vi "Send Update Device Line Configuration.vi"(7 "Message Priority (Normal)":T3=enum."Normal", 8 "error in (no error)":errorcluster, 10 "Line Configuration":T1, 11 "Message Enqueuer":refnum<class "Message Enqueuer.lvclass">) -> (0 "error out":errorcluster, 3 "Message Enqueuer out":refnum<class "Message Enqueuer.lvclass">)   [LabVIEW 2016, in "Optimization Framework.lvlib" / "Update Device Line Configuration Msg.lvclass"]
doc: "This VI sends the message to an actor."
uses:
  Update Device Line Configuration Msg.lvclass
  <vilib>/ActorFramework/Message Enqueuer/Message Enqueuer.lvclass
  <vilib>/ActorFramework/Message Enqueuer/Message Priority.ctl
  Optimization/Controls/Optimization Parameters Line Configuration.ctl
  Optimization/Controls/Optimization Line Configuration Enum.ctl
  C:/Program Files (x86)/National Instruments/LabVIEW 2016/vi.lib/ActorFramework/Message/Message.lvclass
  Update Device Line Configuration Msg.lvclass/Update Device Line Configuration Msg.ctl
  <vilib>/ActorFramework/Message Enqueuer/Message Enqueuer.lvclass/Message Enqueuer.ctl
  <vilib>/ActorFramework/Message Priority Queue/Priority Enqueue.vi
  Optimization/Optimization.lvclass
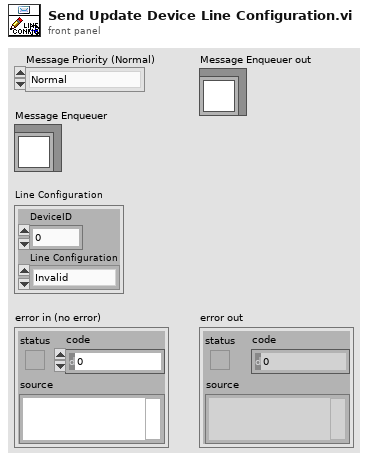
[diagram p1: front panel]
types:
  T1 = typedef "Optimization Framework.lvlib/Optimization.lvclass/Optimization Parameters Line Configuration.ctl" = cluster{"DeviceID":u64, "Line Configuration":T2}
  T2 = typedef "Optimization Framework.lvlib/Optimization.lvclass/Optimization Line Configuration Enum.ctl" = enum8{"Invalid", "L-L", "L-N", "L-G"}
  T3 = typedef "Actor Framework.lvlib/Message Enqueuer.lvclass/Message Priority.ctl" = enum16{"Low", "Normal", "High"}
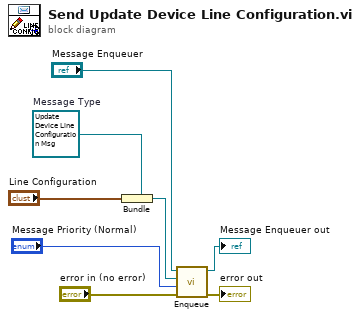
[diagram p0: block diagram]
diagram:
  w5 = refnum<class "Update Device Line Configuration Msg.lvclass"> refnum  # Message Type
  n1 = Bundle(cluster=w5, "Line Configuration") -> (w4:refnum<class "Update Device Line Configuration Msg.lvclass">)
  n2 = call <vilib>:"Enqueue.vi"("error in (no error)"="error in (no error)", "Message Priority (Normal)"="Message Priority (Normal)", "Message"=w4, "Message Enqueuer in"="Message Enqueuer") -> ("error out"=→"error out":errorcluster, "Message Enqueuer out"=→"Message Enqueuer out":refnum<class "Message Enqueuer.lvclass">)  [unwired: 6 in]
